vi "退回.vi"(8 "error in (no error)":errorcluster caption="错误输入（无错误）", 11 "信号数据":dbl[][](array[numeric])) -> (0 "error out":errorcluster caption="错误输出")   [LabVIEW 2015, in "Logging.lvlib"]
uses:
  Logging.lvlib
panel:
  out "右推力最大值":dbl
  out "左右推力差值":dbl
  out "左推力最大值":dbl
  in  "取消按钮":bool
  in  "确定按钮":bool
  # "退回测量结果"
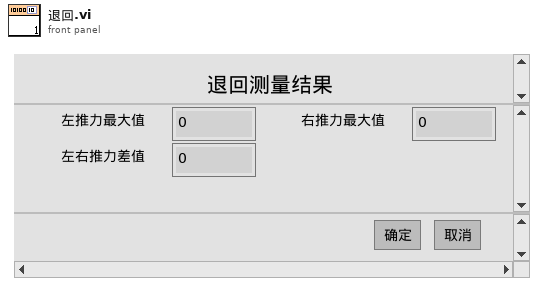
[diagram p1: front panel]
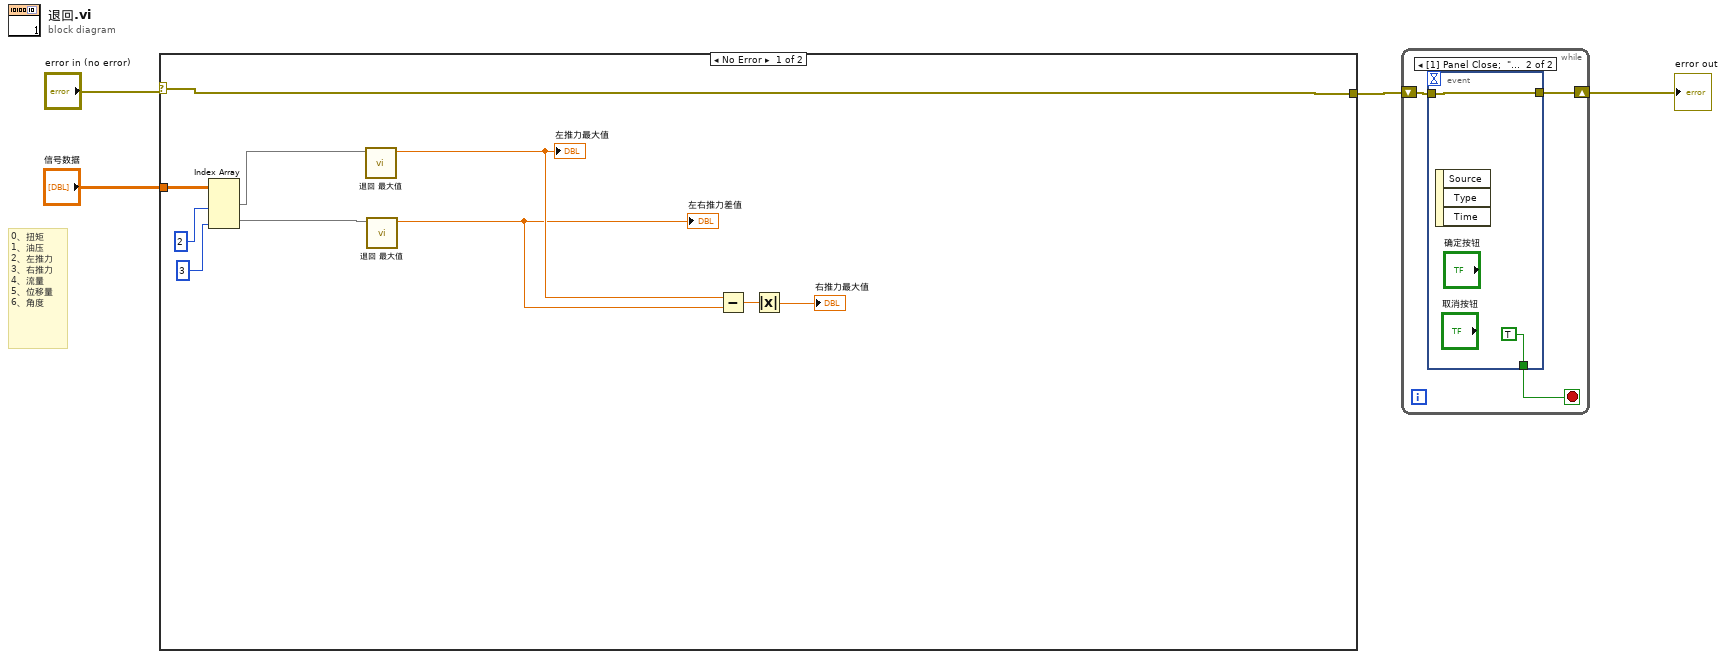
[diagram p0: block diagram]
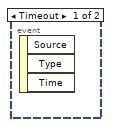
[diagram p2: hidden frame]
diagram:
  # "0、扭矩\n1、油压\n2、左推力\n3、右推力\n4、流量\n5、位移量\n6、角度"
  n1 = case shown="No Error" "error in (no error)" {
    selector: "error in (no error)" -> [w11 w15]
    tunnel: "信号数据" -> [w14 _]
    tunnel: [w11 w15] -> w1
    frame No Error {
      n2 = Index Array(array=w14, index (col) #1=2 ("禁用的索引 (列)"), index (col) #2=3 ("索引 (行)")) -> (element #1=w10:dbl[], element #2=w9:dbl[])  [unwired: 2 in]
      n3 = call "退回 最大值.vi"("推力"=w10) -> ("最大值"=w8:dbl)  [unwired: 10 in]
      "左推力最大值" <- w8
      n4 = call "退回 最大值.vi"("推力"=w9) -> ("最大值"=w7:dbl)  [unwired: 10 in]
      "左右推力差值" <- w7
      n5 = Subtract(x=w8, y=w7) -> (x-y=w13:dbl)
      n6 = Absolute Value(x=w13) -> (abs(x)=→"右推力最大值":dbl)
    }
    frame Error {
    }
  }
  n7 = while {
    shift-right: [w18] -> w2
    shift-left: w1 -> [w17]
    stop <- w16 stop-if-true
    n8 = event shown="[1] Panel Close;  \"确定按钮\", \"取消按钮\": Value Change" {
      selector: _ -> [_ _]
      dyn-events: _ -> [_ _]
      timeout: _ -> [_ _]
      tunnel: [_ w20] -> w18
      tunnel: w17 -> [_ w20]
      tunnel: [_ TRUE] -> w16
      event Timeout {
        n9 = event-data() -> ()  [unwired: 1 in, 3 out]
      }
      event Panel Close; "确定按钮", "取消按钮": Value Change {
        n10 = event-data() -> ()  [unwired: 1 in, 3 out]
      }
    }
  }
  "error out" <- w2
